vi "Press Button.vi"(6 "Standalone?":bool, 7 "Button":T2=enum."SW201 - My Cycle", 8 "Error In":errorcluster, 9 "GEA2 Reference In":refnum<k24>, 10 "GEA Inputs":T1 {"Destination" format="%.0x"; "Source" format="%.0x"}, 11 "Device Selected":i32) -> (0 "Error Out":errorcluster, 1 "GEA2 Reference Out":refnum<k24>)   [LabVIEW 2014]
uses:
  type defs/HEUI Switches.ctl
  Common/LabVIEW GEA2 Toolkit/LabVIEW_GEA2_Toolkit.lvlibp/type defs/Source_Destination.ctl
  Common/LabVIEW GEA2 Toolkit/LabVIEW_GEA2_Toolkit.lvlibp/type defs/ERD Write Data In.ctl
  Common/LabVIEW GEA2 Toolkit/LabVIEW_GEA2_Toolkit.lvlibp/type defs/Data Type.ctl
  C:/Automation/DLLs/PC Dot Net/GeaCommunication.dll
  Common/LabVIEW GEA2 Toolkit/LabVIEW_GEA2_Toolkit.lvlibp
  C:/Automation/DLLs/PC Tools .NET/GeaCommunication.dll
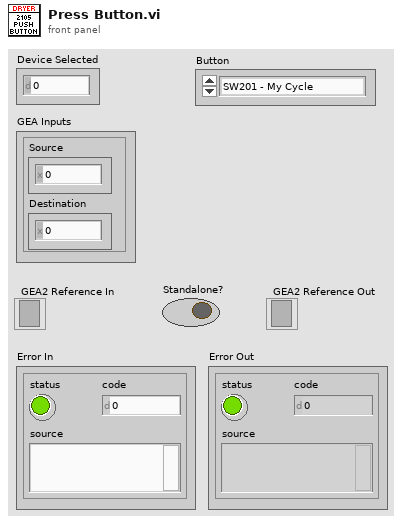
[diagram p1: front panel]
types:
  T1 = typedef "LabVIEW_GEA2_Toolkit.lvlibp/Source_Destination.ctl" = cluster{"Source":u8, "Destination":u8}
  T2 = typedef "HEUI Switches.ctl" = enum16{"Switch Off /  Reset", "SW201 - My Cycle", "SW202 - Delay Dry", "SW203 - Signal / Volume", "SW204 - Damp Alert", "SW205 - Temp", "SW206 - Ext Tumble", "SW207 - Dryness Level", "SW208 -  (-) Time", "SW209 - Time", "SW210 - (+) Time", "SW211 - eDry ", "SW212 - null", "SW213 - Power", "SW214 - Start / Pause"}
  T3 = typedef "LabVIEW_GEA2_Toolkit.lvlibp/ERD Write Data In.ctl" = cluster{"ERD Number":u16, "Data Type":T4, "Data":string}
  T4 = typedef "LabVIEW_GEA2_Toolkit.lvlibp/Data Type.ctl" = enum16{"string", "boolean", "uint8_t", "uint16_t", "uint32_t", "uint64_t", "int8_t", "int16_t", "int32_t", "int64_t"}
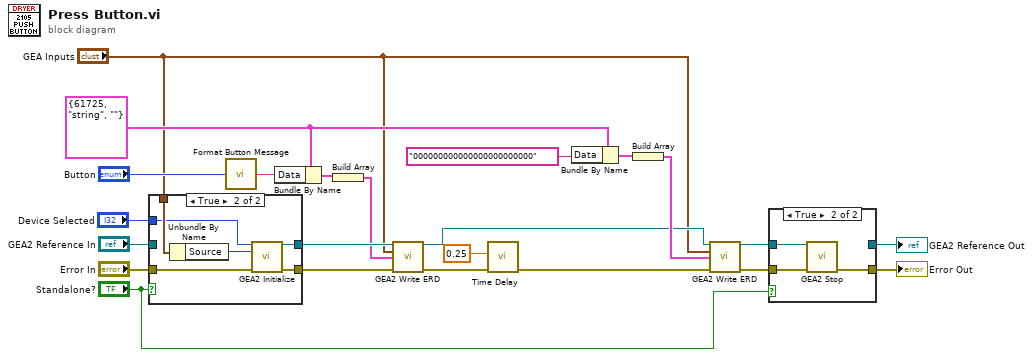
[diagram p0: block diagram]
diagram:
  w3 = T3 {"ERD Number"=61725, "Data Type"=enum."string", "Data"=""} ("ERD Write Data In")
  n1 = case shown="True" "Standalone?" {
    tunnel: "Error In" -> [w24 w31]
    tunnel: [w24 w30] -> w16
    tunnel: "GEA2 Reference In" -> [w25 _]
    tunnel: [w25 w29] -> w14
    tunnel: "GEA Inputs" -> [_ w27]
    tunnel: "Device Selected" -> [_ w26]
    frame False {
    }
    frame True {
      n2 = Unbundle By Name(w27) -> ("Source"=w28:u8)
      n3 = call "GEA2 Initialize.vi"("Board Index"=w26, "Source Address"=w28, "error in"=w31) -> ("GEA2 Reference Out"=w29:refnum<k24>, "error out"=w30:errorcluster)  [unwired: 10 in, 1 out]
    }
  }
  n4 = call "Format Button Message.vi"("Switch"="Button") -> ("Switch Message"=w13:string)  [unwired: 14 in]
  n5 = Bundle By Name(cluster=w3, "Data"=w13) -> (w12:T3)
  n6 = Build Array(w12) -> (w11:T3[])
  n7 = call "GEA2 Write ERD.vi"("GEA2 Reference In"=w14, "GEA Inputs"="GEA Inputs", "Write ERD List"=w11, "Error In"=w16) -> ("GEA2 Reference Out"=w4:refnum<k24>, "Error Out"=w15:errorcluster)  [unwired: 9 in, 1 out]
  n8 = call "Time Delay"("error in (no error)"=w15, "Delay Time (s)"=0.25) -> ("error out"=w9:errorcluster)  [unwired: 9 in]
  n9 = Bundle By Name(cluster=w3, "Data"="000000000000000000000000" ("Message")) -> (w6:T3)
  n10 = Build Array(w6) -> (w5:T3[])
  n11 = call "GEA2 Write ERD.vi"("GEA2 Reference In"=w4, "GEA Inputs"="GEA Inputs", "Write ERD List"=w5, "Error In"=w9) -> ("GEA2 Reference Out"=w10:refnum<k24>, "Error Out"=w8:errorcluster)  [unwired: 9 in, 1 out]
  n12 = case shown="True" "Standalone?" {
    tunnel: [w32 w36] -> w19
    tunnel: w10 -> [w33 w35]
    tunnel: [w33 _] -> w18
    tunnel: w8 -> [w32 w34]
    frame False {
    }
    frame True {
      n13 = call "GEA2 Stop.vi"("GEA2 Reference In"=w35, "Error In"=w34) -> ("Error Out"=w36:errorcluster)  [unwired: 13 in]
    }
  }
  "Error Out" <- w19
  "GEA2 Reference Out" <- w18
